vi "load method in to cache.vi"(8 "error in (no error)":errorcluster, 10 "method name":string, 11 "Method Manager in":refnum<class "Method Loader.lvclass">) -> (0 "error out":errorcluster, 2 "found?":bool, 3 "Method Manager out":refnum<class "Method Loader.lvclass">)   [LabVIEW 2020, in "JSON-RPC Lib.lvlib" / "Method Loader.lvclass"]
uses:
  Method Loader.lvclass
  method type.ctl
  Method Loader.lvclass/Method Loader.ctl
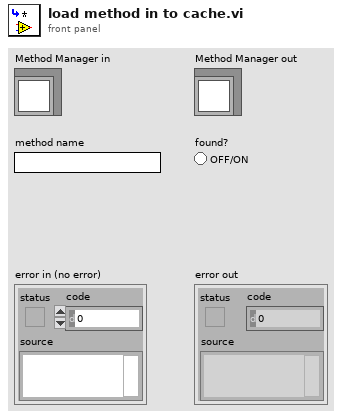
[diagram p1: front panel]
types:
  T1 = typedef "JSON-RPC Lib.lvlib/Method Loader.lvclass/method type.ctl" = refnum<vi>
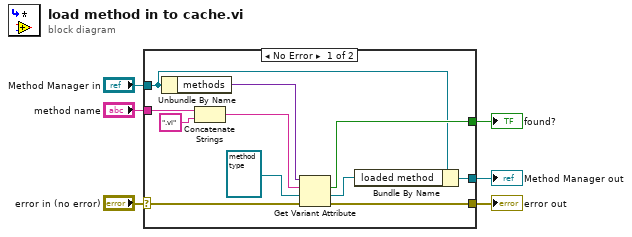
[diagram p0: block diagram]
diagram:
  n1 = case shown="No Error" "error in (no error)" {
    selector: "error in (no error)" -> [w14 w19]
    tunnel: [w16 w19] -> w3
    tunnel: [w15 _] -> w6
    tunnel: "method name" -> [w12 _]
    tunnel: "Method Manager in" -> [w8 w18]
    tunnel: [w10 w18] -> w1
    frame No Error {
      n2 = Unbundle By Name(w8) -> ("methods"=w9:variant)
      n3 = Concatenate Strings(w12, ".vi" ("string")) -> (w17:string)
      n4 = Get Variant Attribute(Variant=w9, name=w17, default value (empty Variant)=T1 refnum ("type specifier VI Refnum (for type only)"), error in=w14) -> (found=w15:bool, value=w11:T1, error out=w16:errorcluster)  [unwired: 1 out]
      n5 = Bundle By Name(cluster=w8, "loaded method"=w11) -> (w10:refnum<class "Method Loader.lvclass">)
    }
    frame Error {
    }
  }
  "error out" <- w3
  "Method Manager out" <- w1
  "found?" <- w6
